vi "GetSensorData.vi"(11 "Sensor Sessions":T4) -> (0 "Obstacles":T3, 2 "Pose":T5, 3 "Sessions Out":T2)   [LabVIEW 2011]
uses:
  <vilib>/vision/Image Controls.llb/IMAQ Image.ctl
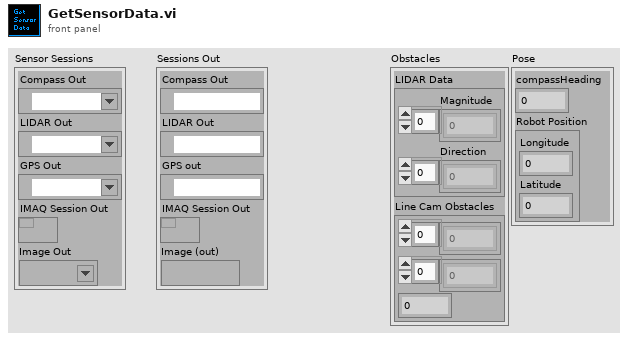
[diagram p1: front panel]
types:
  T1 = typedef "IMAQ Image.ctl" = refnum<image>
  T2 = cluster{"Compass Out":refnum<visa-resource-name>, "LIDAR Out":refnum<visa-resource-name>, "GPS out":refnum<visa-resource-name>, "IMAQ Session Out":refnum<k11>, "Image (out)":T1}
  T3 = cluster{"LIDAR Data":cluster{"Magnitude":dbl[], "Direction":dbl[]}, "Line Cam Obstacles":cluster{dbl[], dbl[], i32}}
  T4 = cluster{"Compass Out":refnum<visa-resource-name>, "LIDAR Out":refnum<visa-resource-name>, "GPS Out":refnum<visa-resource-name>, "IMAQ Session Out":refnum<k11>, "Image Out":T1}
  T5 = cluster{"compassHeading":dbl, "Robot Position":cluster{"Longitude":dbl, "Latitude":dbl}}
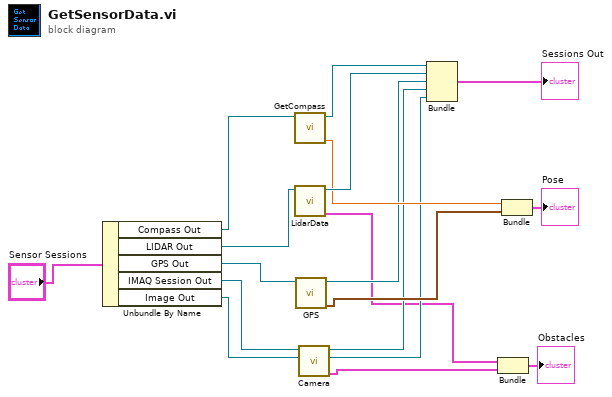
[diagram p0: block diagram]
diagram:
  n1 = Unbundle By Name("Sensor Sessions") -> ("Compass Out"=w12:refnum<visa-resource-name>, "LIDAR Out"=w11:refnum<visa-resource-name>, "GPS Out"=w10:refnum<visa-resource-name>, "IMAQ Session Out"=w8:refnum<k11>, "Image Out"=w7:T1)
  n2 = call "GetCompass.vi"("Compass In"=w12) -> ("compassHeading"=w15:dbl, "Compass Out"=w18:refnum<visa-resource-name>)  [unwired: 9 in]
  n3 = call "LidarData.vi"("LIDAR IN"=w11) -> ("LIDAR Data"=w4:cluster{"Magnitude":dbl[], "Direction":dbl[]}, "LIDAR Out"=w17:refnum<visa-resource-name>)  [unwired: 9 in]
  n4 = call "GPS.vi"("GPS In"=w10) -> ("Robot Position"=w16:cluster{"Longitude":dbl, "Latitude":dbl}, "GPS out"=w9:refnum<visa-resource-name>)  [unwired: 7 in]
  n5 = call "Camera.vi"("Image In"=w7, "IMAQ Session In"=w8) -> ("Line Cam Obstacles"=w3:cluster{dbl[], dbl[], i32}, "Image (out)"=w5:T1, "IMAQ Session Out"=w6:refnum<k11>)  [unwired: 7 in]
  n6 = Bundle("Compass Out"=w18, "LIDAR Out"=w17, "GPS out"=w9, "IMAQ Session Out"=w6, "Image (out)"=w5) -> (→"Sessions Out":T2)  [unwired: 1 in]
  n7 = Bundle("LIDAR Data"=w4, "Line Cam Obstacles"=w3) -> (→"Obstacles":T3)  [unwired: 1 in]
  n8 = Bundle("compassHeading"=w15, "Robot Position"=w16) -> (→"Pose":T5)  [unwired: 1 in]
